vi "AY.vi"(6 "时间值":i16, 8 "数值":i16, 9 "width":i32[](array[numeric]), 10 "begin":i32[](array[numeric]), 11 "act":bool[](array[boolean])) -> (2 "布尔":bool)   [LabVIEW 2018]
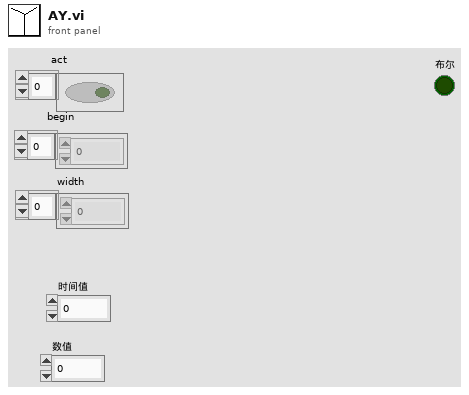
[diagram p1: front panel]
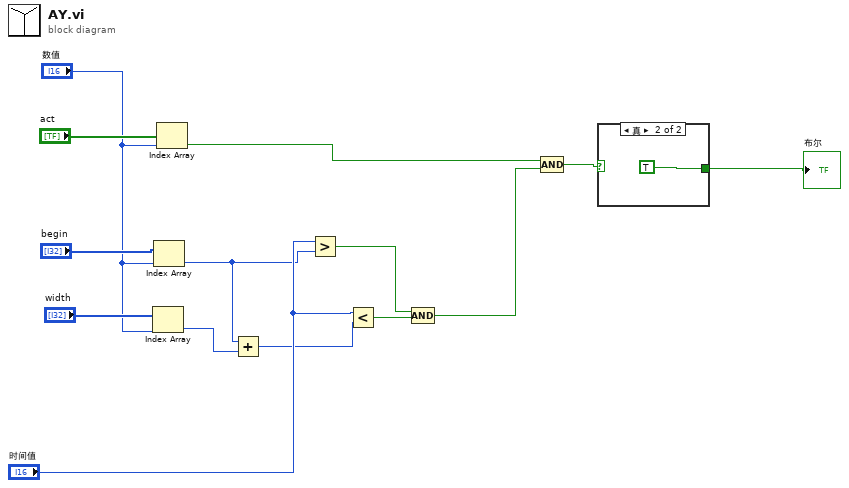
[diagram p0: block diagram]
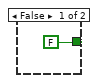
[diagram p2: hidden frame]
diagram:
  n1 = Index Array(array="width", index="数值") -> (element=w8:i32)
  n2 = Index Array(array="begin", index="数值") -> (element=w9:i32)
  n3 = Index Array(array="act", index="数值") -> (element=w1:bool)
  n4 = Add(x=w9, y=w8) -> (x+y=w10:i32)
  n5 = Greater?(x="时间值", y=w9) -> (0:w7:bool)
  n6 = Less?(x="时间值", y=w10) -> (x < y?=w6:bool)
  n7 = Compound Arithmetic op=AND ("复合运算")(w7, w6) -> (w5:bool)
  n8 = Compound Arithmetic op=AND ("复合运算")(w1, w5) -> (w4:bool)
  n9 = case shown="真" w4 {
    tunnel: [FALSE TRUE] -> w3
    frame False {
    }
    frame True {
    }
  }
  "布尔" <- w3
